vi "Add to Tree (Internal).vi"(4 "Child Tag":string, 5 "Child Position":i32, 6 "Display Text Override":string, 7 "Add children? (T)":bool=TRUE, 8 "error in (no error)":errorcluster, 9 "Parent Tag":string, 10 "Tree Manager in":refnum<class "Tree Manager.lvclass">, 11 "Data Item in":refnum<class "Data Item.lvclass">) -> (0 "error out":errorcluster, 1 "New Tag":string, 2 "Tree Manager out":refnum<class "Tree Manager.lvclass">, 3 "Data Item out":refnum<class "Data Item.lvclass">)   [LabVIEW 2026, in "VILab.lvlib" / "Data Item.lvclass"]
uses:
  Data Item.lvclass
  Tree Manager/Tree Manager.lvclass
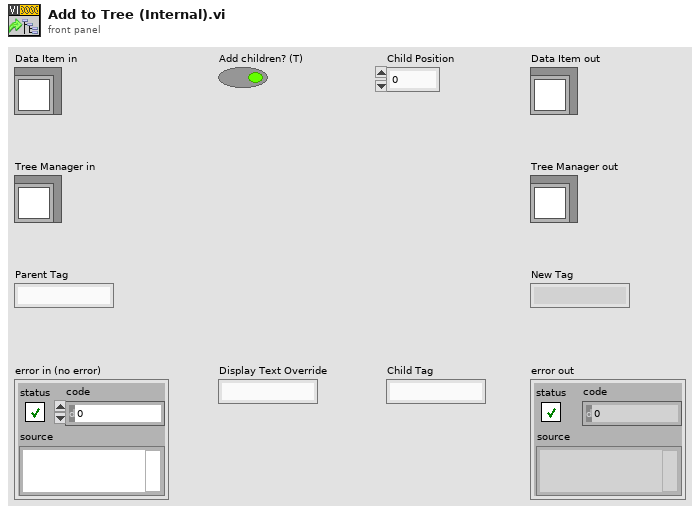
[diagram p1: front panel]
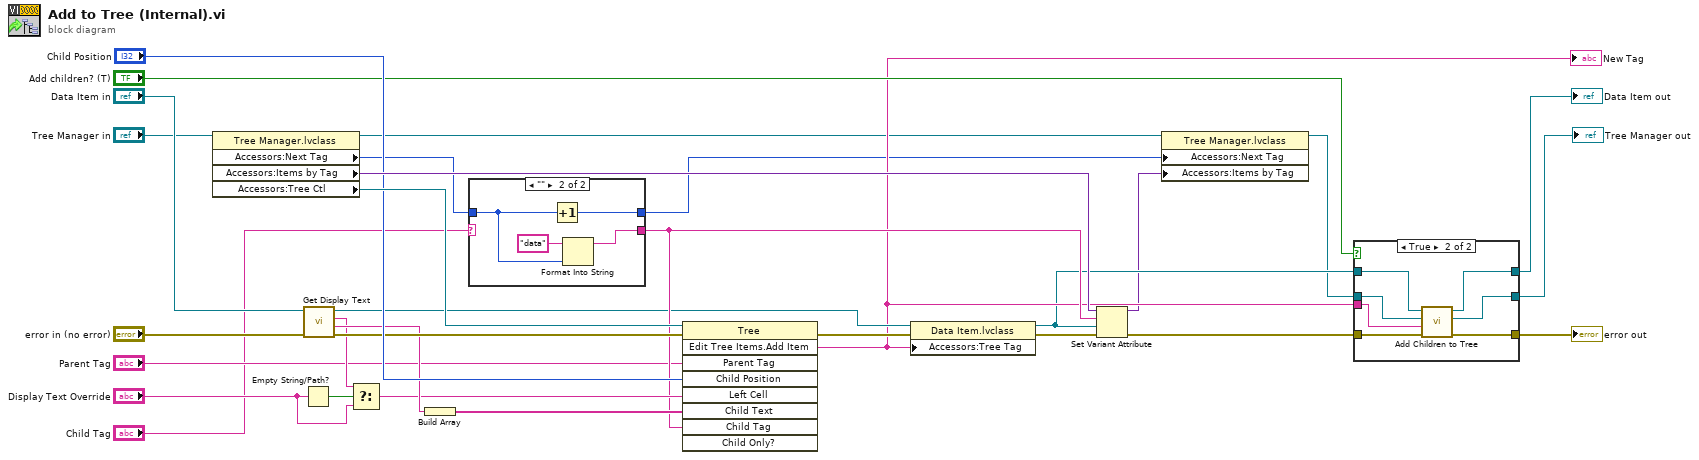
[diagram p0: block diagram]
diagram:
  n1 = property class="Tree Manager.lvclass"(reference="Tree Manager in") -> (reference out=w4:refnum<class "Tree Manager.lvclass">, "Accessors:Next Tag"=w1:u64, "Accessors:Items by Tag"=w29:variant, "Accessors:Tree Ctl"=w30:refnum<vi>)  [unwired: 1 in, 1 out]
  n2 = Empty String/Path?(string/path="Display Text Override") -> (empty?=w21:bool)
  n3 = call-dynamic "Get Display Text.vi"("error in (no error)"="error in (no error)", "Data Item in"="Data Item in") -> ("error out"=w27:errorcluster, "Detail Text"=w26:string, "Display Name"=w22:string, "Data Item out"=w18:refnum<class "Data Item.lvclass">)  [unwired: 6 in]
  n4 = Select(t=w22, s=w21, f="Display Text Override") -> (s? t:f=w24:string)
  n5 = Build Array(w26) -> (w25:string[])
  n6 = case shown="\"\"" "Child Tag" {
    selector: "Child Tag" -> [w31 _]
    tunnel: [w31 w35] -> w23
    tunnel: [w32 w34] -> w3
    tunnel: w1 -> [w32 w33]
    frame Default {
    }
    frame "" {
      n7 = Increment(x=w33) -> (x+1=w34:u64)
      n8 = Format Into String(initial string="data", w33) -> (resulting string=w35:string)  [unwired: 2 in, 1 out]
    }
  }
  n9 = invoke class="Tree" method="Edit Tree Items.Add Item"(reference=w30, error in=w27, "Parent Tag"="Parent Tag", "Child Position"="Child Position", "Left Cell"=w24, "Child Text"=w25, "Child Tag"=w23) -> (error out=w20:errorcluster, "Edit Tree Items:Add Item"=w10:string)  [unwired: 2 in, 7 out]
  "New Tag" <- w10
  n10 = property class="Data Item.lvclass"(reference=w18, error in=w20, "Accessors:Tree Tag"=w10) -> (reference out=w9:refnum<class "Data Item.lvclass">, error out=w19:errorcluster)
  n11 = Set Variant Attribute(Variant=w29, name=w23, value=w9) -> (Variant out=w5:variant)  [unwired: 1 in, 2 out]
  n12 = property class="Tree Manager.lvclass"(reference=w4, "Accessors:Next Tag"=w3, "Accessors:Items by Tag"=w5) -> (reference out=w8:refnum<class "Tree Manager.lvclass">)  [unwired: 1 in, 1 out]
  n13 = case shown="True" "Add children? (T)" {
    tunnel: w8 -> [w38 w46]
    tunnel: w19 -> [w37 w44]
    tunnel: w10 -> [_ w45]
    tunnel: [w38 w42] -> w6
    tunnel: w9 -> [w39 w40]
    tunnel: [w39 w43] -> w11
    tunnel: [w37 w41] -> w7
    frame False {
    }
    frame True {
      n14 = call "Add Children to Tree.vi"("error in (no error)"=w44, "Parent Tag"=w45, "Tree Manager in"=w46, "Data Item in"=w40) -> ("error out"=w41:errorcluster, "Tree Manager out"=w42:refnum<class "Tree Manager.lvclass">, "Data Item out"=w43:refnum<class "Data Item.lvclass">)  [unwired: 5 in]
    }
  }
  "error out" <- w7
  "Data Item out" <- w11
  "Tree Manager out" <- w6
